vi "ReadTestItems.vi"(8 "error in (no error)":errorcluster caption="错误输入（无错误）", 11 "产品型号":refnum<vi>) -> (0 "error out":errorcluster, 4 "data":string[](array[string]))   [LabVIEW 2013]
uses:
  <vilib>/Utility/NIReport.llb/NI_report.lvclass
  SourceCode/GlobalValue.vi
  <vilib>/addons/_office/excel.llb/Excel Get Data ([str]).vi
  <vilib>/addons/_office/NI_ReportGenerationToolkit.lvlib
  <vilib>/Utility/NIReport.llb/Excel/NI_Excel.lvclass
panel:
  out "已删除元素的数组子集":string[][](array[string])
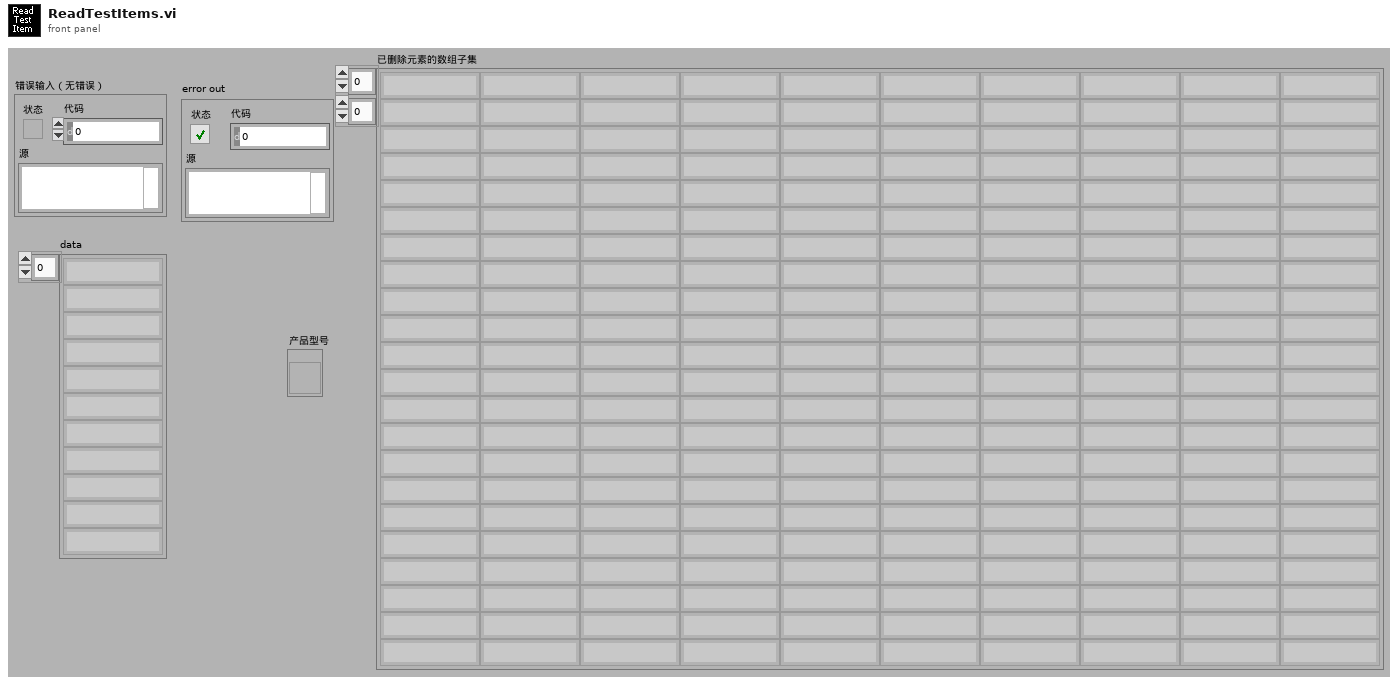
[diagram p1: front panel]
types:
  T1 = enum16{"maximized", "minimized", "normal", "no change"}
  T2 = enum16{"Standard Report", "HTML", "Word", "Excel"}
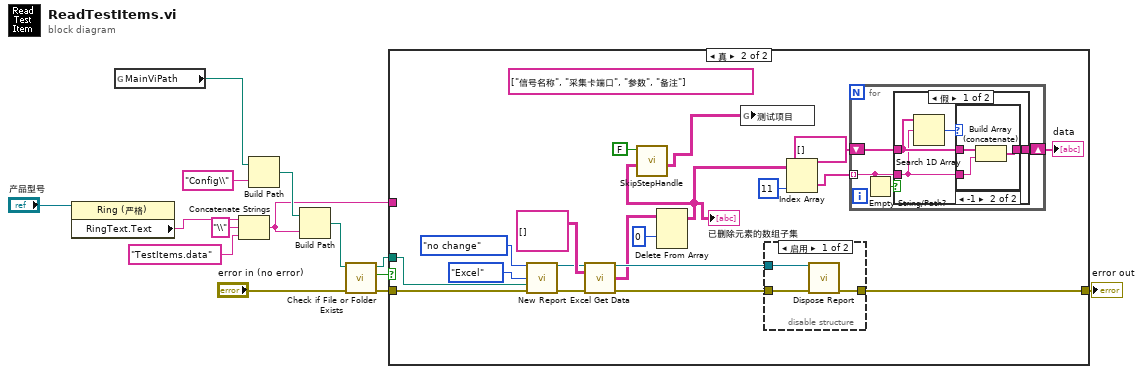
[diagram p0: block diagram]
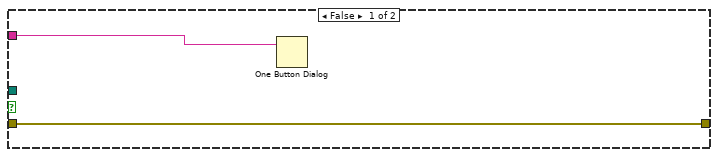
[diagram p2: hidden frame]
diagram:
  n1 = property on="属性节点" class="Ring (严格)"(reference="产品型号") -> ("RingText.Text"=w2:string)  [unwired: 1 in, 2 out]
  n2 = global read "GlobalValue.vi" "MainViPath"() -> (w3:path)
  n3 = Concatenate Strings(w2, "\\" ("字符串"), "TestItems.data" ("字符串")) -> (w4:string)
  n4 = Build Path(base path=w3, name or relative path="Config\\" ("字符串")) -> (appended path=w8:path)
  n5 = Build Path(base path=w8, name or relative path=w4) -> (appended path=w11:path)
  n6 = call <vilib>:"Check if File or Folder Exists.vi"("error in (no error)"="error in (no error)", "path"=w11) -> ("error out"=w10:errorcluster, "file or folder exists?"=w13:bool, "dup path"=w12:path)  [unwired: 7 out]
  n7 = case shown="真" w13 {
    tunnel: w10 -> [w16 w34]
    tunnel: w12 -> [_ w35]
    tunnel: [w16 w32] -> w7
    tunnel: w4 -> [w15 _]
    frame False {
      n8 = One Button Dialog(message=w15) -> ()  [unwired: 1 in, 1 out]
    }
    frame True {
      (unwired) string[] ["信号名称", "采集卡端口", "参数", "备注"] ("已删除的部分")
      n9 = call <vilib>:"New Report.vi"("window state (normal)"=T1."no change", "report type"=T2."Excel", "template (empty)"=w35, "error in (no error)"=w34) -> ("report out"=w29:refnum<class "NI_report.lvclass">, "error out"=w28:errorcluster)  [unwired: 2 in, 8 out]
      n10 = call-poly <vilib>:"Excel Get Data.vi"("report in"=w29, "data type"=string[][] [], "error in (no error)"=w28) -> ("report out"=w33:refnum<class "NI_report.lvclass">, "data"=w27:string[][], "error out"=w24:errorcluster)  [unwired: 10 in]
      n11 = Delete From Array(array=w27, index (row)=0 ("索引 (行)")) -> (array with subset deleted=w17:string[][])  [unwired: 2 in, 1 out]
      "已删除元素的数组子集" <- w17
      n12 = call "SkipStepHandle.vi"("ItemNamesIn"=w17, "ShowSkipStep?"=FALSE) -> ("ItemNamesOut"=w22:string[][])  [unwired: 9 in]
      n13 = global write "GlobalValue.vi" "测试项目"(w22) -> ()
      n14 = disable-structure shown="启用" {
        disable-tunnel: w33 -> [w51 _]
        disable-tunnel: [w50 _] -> w32
        disable-tunnel: w24 -> [w49 _]
        frame Enabled {
          n15 = call-dynamic "Dispose Report.vi"("report in"=w51, "error in (no error)"=w49) -> ("error out"=w50:errorcluster)  [unwired: 3 in, 10 out]
        }
        frame Disabled {
        }
      }
      n16 = Index Array(array=w17, index (col)=11 ("禁用的索引 (列)")) -> (element=w21:string[])  [unwired: 1 in]
      n17 = for "For循环" {
        shift-right: [w38] -> w18
        shift-left: string[] [] -> [w39]
        tunnel: w21 -> [w37] mode=indexing
        n18 = Empty String/Path?(string/path=w37) -> (empty?=w36:bool)
        n19 = case shown="假" w36 {
          tunnel: w39 -> [w42 w48]
          tunnel: [w41 w48] -> w38
          tunnel: w37 -> [w40 _]
          frame False {
            n20 = Search 1D Array(1D array=w42, element=w40) -> (index of element=w43:i32)  [unwired: 1 in]
            n21 = case shown="-1" w43 {
              tunnel: w42 -> [w44 w46]
              tunnel: [w44 w45] -> w41
              tunnel: w40 -> [_ w47]
              frame 1, Default {
              }
              frame -1 {
                n22 = Build Array (concatenate)(w46, w47) -> (w45:string[])
              }
            }
          }
          frame True {
          }
        }
      }
      "data" <- w18
    }
  }
  "error out" <- w7
